vi "To Variant.vi"(0 "Obj in":refnum<class "FM Sweep.lvclass">, 11 "error in (no error)":errorcluster) -> (4 "Obj out":refnum<class "FM Sweep.lvclass">, 8 "Array":variant[](array[variant]), 15 "error out":errorcluster)   [LabVIEW 2020, in "FM Sweep.lvclass"]
uses:
  FM Sweep.lvclass
  FM Sweep.lvclass/FM Sweep.ctl
  Waveform/Waveform.lvclass
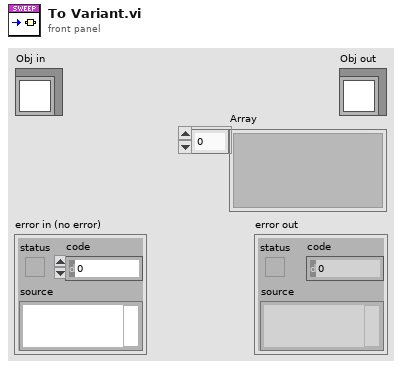
[diagram p1: front panel]
types:
  T1 = typedef "FM Sweep.lvclass/Serialized.ctl" = cluster{"Rate":dbl, "Fmin (Hz)":dbl, "Fmax (Hz)":dbl, "Linear":bool, "ConstFreqRamp":bool}
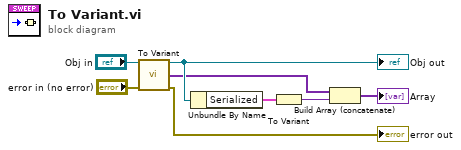
[diagram p0: block diagram]
diagram:
  n1 = call-parent "To Variant.vi"("Obj in"="Obj in", "error in (no error)"="error in (no error)") -> ("Obj out"=w3:refnum<class "FM Sweep.lvclass">, "Array"=w2:variant[], "error out"=→"error out":errorcluster)  [unwired: 11 in]
  "Obj out" <- w3
  n2 = Unbundle By Name(w3) -> ("Serialized"=w4:T1)
  n3 = To Variant(anything=w4) -> (Variant=w5:variant)
  n4 = Build Array (concatenate)(w2, w5) -> (→"Array":variant[])
